vi "Launch Action - XNET CAN Readers.vi"(8 "error in (no error)":errorcluster, 11 "CAN Configurations":T1[](array[typedef]) {"Sample Rate (Hz)" format="%#_13g"}) -> (0 "error out":errorcluster)   [LabVIEW 2021, in "XNET-CAN-Signal-Logger.lvlib"]
uses:
  XNET-CAN-Signal-Logger.lvlib
  Typedef/Def-CAN Port Configuration.ctl
  Action - XNET CAN Reader.vi
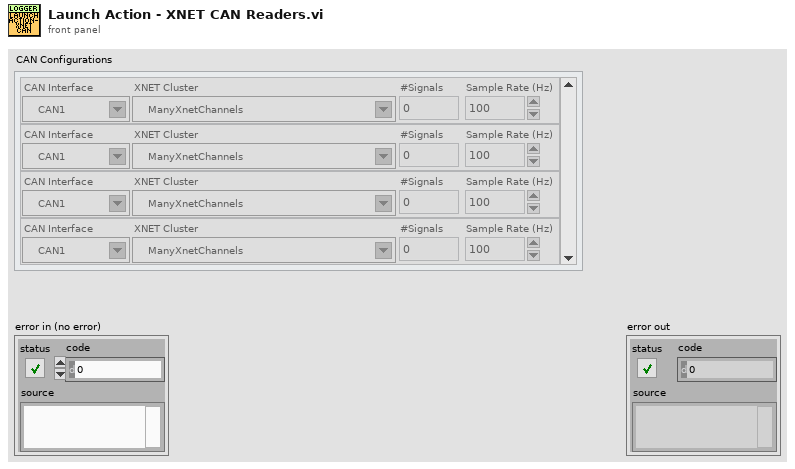
[diagram p1: front panel]
types:
  T1 = typedef "XNET-CAN-Signal-Logger.lvlib/Def-CAN Port Configuration.ctl" = cluster{"CAN Interface":refnum<k21>, "XNET Cluster":refnum<k21>, "#Signals":i32, "Sample Rate (Hz)":dbl}
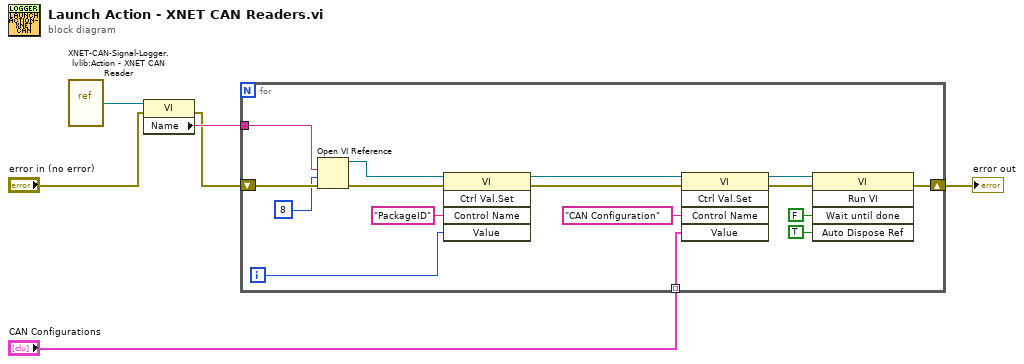
[diagram p0: block diagram]
diagram:
  n1 = vi-ref "XNET-CAN-Signal-Logger.lvlib:Action - XNET CAN Reader.vi"() -> (w6:refnum<vi>)
  n2 = property class="VI"(reference=w6, error in="error in (no error)") -> (error out=w3:errorcluster, "Name"=w5:string)  [unwired: 1 out]
  n3 = for {
    tunnel: w5 -> [w22]
    shift-right: [w15] -> w2
    shift-left: w3 -> [w20]
    tunnel: "CAN Configurations" -> [w9] mode=indexing
    i -> [w8]
    n4 = Open VI Reference(vi path=w22, options=8, error in (no error)=w20) -> (vi reference=w12:refnum<vi>, error out=w13:errorcluster)  [unwired: 3 in]
    n5 = invoke class="VI" method="Ctrl Val.Set"(reference=w12, error in=w13, "Control Name"="PackageID", "Value"=w8) -> (reference out=w11:refnum<vi>, error out=w10:errorcluster)  [unwired: 1 in, 3 out]
    n6 = invoke class="VI" method="Ctrl Val.Set"(reference=w11, error in=w10, "Control Name"="CAN Configuration", "Value"=w9) -> (reference out=w19:refnum<vi>, error out=w18:errorcluster)  [unwired: 1 in, 3 out]
    n7 = invoke class="VI" method="Run VI"(reference=w19, error in=w18, "Wait until done"=FALSE ("Wait Until Done"), "Auto Dispose Ref"=TRUE ("Auto Dispose Reference")) -> (error out=w15:errorcluster)  [unwired: 1 in, 4 out]
  }
  "error out" <- w2
